vi "targetRangeSignCorrection.vi"(4 "Current Ramp Position":i16, 5 "increment_x":i16, 6 "target":i16, 7 "Ramp range":cluster{"min_x":i16, "max_x":i16}) -> (1 "Increment corrected for direction":i16, 2 "position not reached":bool, 3 "CorrectedTarget":i16)   [LabVIEW 2016]
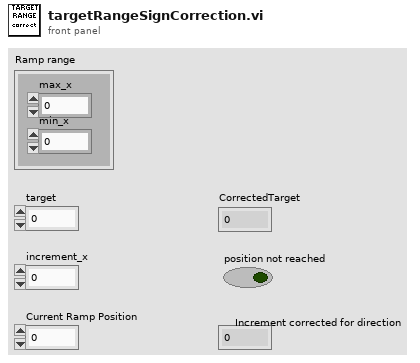
[diagram p1: front panel]
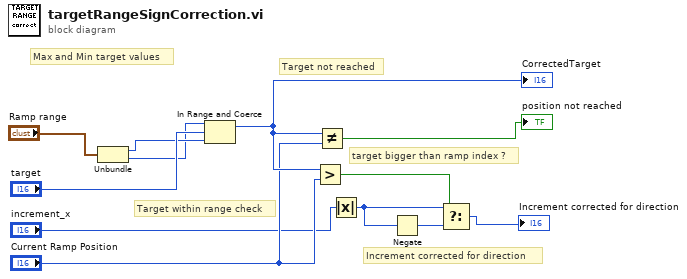
[diagram p0: block diagram]
diagram:
  # "Max and Min target values"
  # "Increment corrected for direction"
  # "target bigger than ramp index ?"
  # "Target not reached"
  # "Target within range check"
  n1 = Unbundle("Ramp range") -> ("min_x"=w2:i16, "max_x"=w1:i16)
  n2 = In Range and Coerce(upper limit=w1, x="target", lower limit=w2) -> (coerced(x)=w8:i16)  [unwired: 1 out]
  "CorrectedTarget" <- w8
  n3 = Greater?(x=w8, y="Current Ramp Position") -> (0:w10:bool)
  n4 = Not Equal?(x=w8, y="Current Ramp Position") -> (x != y?=→"position not reached":bool)
  n5 = Absolute Value(x="increment_x") -> (abs(x)=w12:i16)
  n6 = Negate(x=w12) -> (-x=w11:i16)
  n7 = Select(t=w12, s=w10, f=w11) -> (s? t:f=→"Increment corrected for direction":i16)
